vi "Destroy.vi"(8 "error in (no error)":errorcluster, 11 "TDMS Sink in":refnum<class "TDMS Sink.lvclass">) -> (0 "error out":errorcluster)   [LabVIEW 2020, in "LV Log.lvlib" / "TDMS Sink.lvclass"]
uses:
  TDMS Sink.lvclass
  TDMS Sink.lvclass/TDMS Sink.ctl
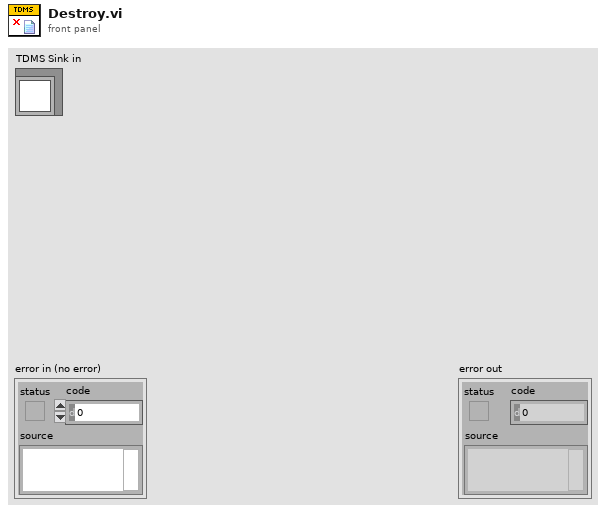
[diagram p1: front panel]
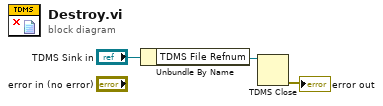
[diagram p0: block diagram]
diagram:
  n1 = Unbundle By Name("TDMS Sink in") -> ("TDMS File Refnum"=w1:refnum<k34>)
  n2 = TDMS Close(11:w1) -> (0:→"error out":errorcluster)  [unwired: 1 in, 1 out]
